vi "Register Step Handler.vi"(8 "error in (no error)":errorcluster, 10 "Handler":refnum<class "Handler.lvclass">, 11 "Server in":refnum<class "Server.lvclass">) -> (0 "error out":errorcluster, 3 "Server out":refnum<class "Server.lvclass">)   [LabVIEW 2020, in "HTTP Server.lvlib" / "Server.lvclass"]
uses:
  Server.lvclass
  Handler/Handler.lvclass
  Server.lvclass/Server.ctl
  Connection Handler/Connection Handler.lvclass
  Request Handler/Request Handler.lvclass
  Route Handler/Route Handler.lvclass
  Controller Handler/Controller Handler.lvclass
  Controller/Controller.lvclass
  Response Handler/Response Handler.lvclass
  Complete Handler/Complete Handler.lvclass
  Exception Handler/Exception Handler.lvclass
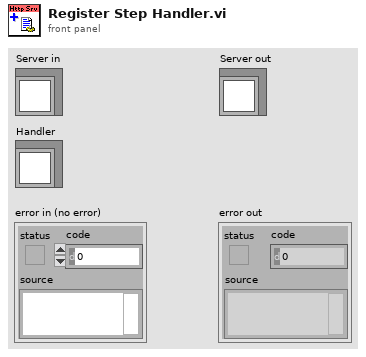
[diagram p1: front panel]
types:
  T1 = typedef "HTTP Server.lvlib/Processing Step.ctl" = enum16{"Connection", "Request", "Routing", "Controller Init", "Controller", "Response", "Cleanup", "Exception"}
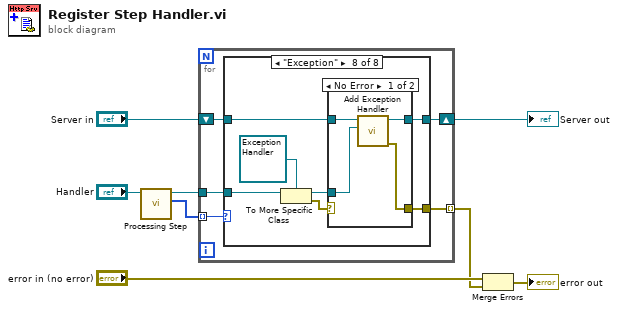
[diagram p0: block diagram]
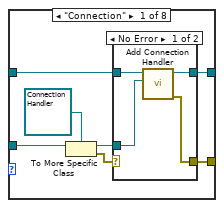
[diagram p2: hidden frame]
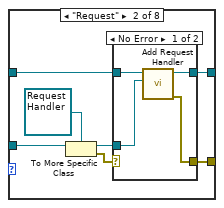
[diagram p4: hidden frame]
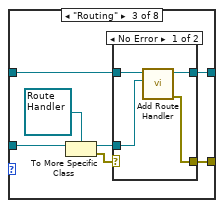
[diagram p6: hidden frame]
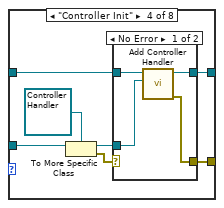
[diagram p8: hidden frame]
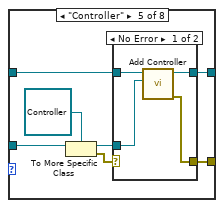
[diagram p10: hidden frame]
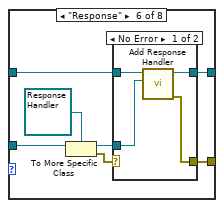
[diagram p12: hidden frame]
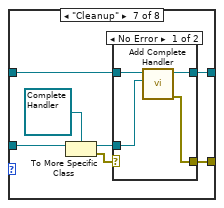
[diagram p14: hidden frame]
diagram:
  n1 = call-dynamic "Processing Step.vi"("Handler in"="Handler") -> ("Array"=w5:T1[], "Handler out"=w4:refnum<class "Handler.lvclass">)  [unwired: 8 in, 1 out]
  n2 = for {
    tunnel: w5 -> [w13] mode=indexing
    tunnel: w4 -> [w11]
    shift-right: [w10] -> w2
    shift-left: "Server in" -> [w12]
    tunnel: [w9] -> w1 mode=indexing
    n3 = case shown="\"Exception\"" w13 {
      tunnel: w12 -> [w16 w29 w42 w55 w68 w81 w94 w107]
      tunnel: w11 -> [w20 w33 w46 w59 w72 w85 w98 w111]
      tunnel: [w15 w28 w41 w54 w67 w80 w93 w106] -> w10
      tunnel: [w14 w27 w40 w53 w66 w79 w92 w105] -> w9
      frame "Connection" {
        n4 = To More Specific Class(target class=refnum<class "Connection Handler.lvclass"> refnum ("HTTP Server.lvlib:Connection Handler.lvclass"), reference=w20) -> (specific class reference=w18:refnum<class "Connection Handler.lvclass">, error out=w17:errorcluster)  [unwired: 1 in]
        n5 = case shown="No Error" w17 {
          selector: w17 -> [_ w26]
          tunnel: w18 -> [w23 _]
          tunnel: w16 -> [w24 w25]
          tunnel: [w22 w25] -> w15
          tunnel: [w21 w26] -> w14
          frame No Error {
            n6 = call "Add Connection Handler.vi"("Connection Handler"=w23, "Server in"=w24) -> ("error out"=w21:errorcluster, "Server out"=w22:refnum<class "Server.lvclass">)  [unwired: 8 in]
          }
          frame Error {
          }
        }
      }
      frame "Request" {
        n7 = To More Specific Class(target class=refnum<class "Request Handler.lvclass"> refnum ("HTTP Server.lvlib:Request Handler.lvclass"), reference=w33) -> (specific class reference=w31:refnum<class "Request Handler.lvclass">, error out=w30:errorcluster)  [unwired: 1 in]
        n8 = case shown="No Error" w30 {
          selector: w30 -> [_ w39]
          tunnel: w31 -> [w36 _]
          tunnel: w29 -> [w37 w38]
          tunnel: [w35 w38] -> w28
          tunnel: [w34 w39] -> w27
          frame No Error {
            n9 = call "Add Request Handler.vi"("Request Handler"=w36, "Server in"=w37) -> ("error out"=w34:errorcluster, "Server out"=w35:refnum<class "Server.lvclass">)  [unwired: 8 in]
          }
          frame Error {
          }
        }
      }
      frame "Routing" {
        n10 = To More Specific Class(target class=refnum<class "Route Handler.lvclass"> refnum ("HTTP Server.lvlib:Route Handler.lvclass"), reference=w46) -> (specific class reference=w44:refnum<class "Route Handler.lvclass">, error out=w43:errorcluster)  [unwired: 1 in]
        n11 = case shown="No Error" w43 {
          selector: w43 -> [_ w52]
          tunnel: w44 -> [w49 _]
          tunnel: w42 -> [w50 w51]
          tunnel: [w48 w51] -> w41
          tunnel: [w47 w52] -> w40
          frame No Error {
            n12 = call "Add Route Handler.vi"("Route Handler"=w49, "Server in"=w50) -> ("error out"=w47:errorcluster, "Server out"=w48:refnum<class "Server.lvclass">)  [unwired: 8 in]
          }
          frame Error {
          }
        }
      }
      frame "Controller Init" {
        n13 = To More Specific Class(target class=refnum<class "Controller Handler.lvclass"> refnum ("HTTP Server.lvlib:Controller Handler.lvclass"), reference=w59) -> (specific class reference=w57:refnum<class "Controller Handler.lvclass">, error out=w56:errorcluster)  [unwired: 1 in]
        n14 = case shown="No Error" w56 {
          selector: w56 -> [_ w65]
          tunnel: w57 -> [w62 _]
          tunnel: w55 -> [w63 w64]
          tunnel: [w61 w64] -> w54
          tunnel: [w60 w65] -> w53
          frame No Error {
            n15 = call "Add Controller Handler.vi"("Controller Handler"=w62, "Server in"=w63) -> ("error out"=w60:errorcluster, "Server out"=w61:refnum<class "Server.lvclass">)  [unwired: 8 in]
          }
          frame Error {
          }
        }
      }
      frame "Controller" {
        n16 = To More Specific Class(target class=refnum<class "Controller.lvclass"> refnum ("HTTP Server.lvlib:Controller.lvclass"), reference=w72) -> (specific class reference=w70:refnum<class "Controller.lvclass">, error out=w69:errorcluster)  [unwired: 1 in]
        n17 = case shown="No Error" w69 {
          selector: w69 -> [_ w78]
          tunnel: w70 -> [w75 _]
          tunnel: w68 -> [w76 w77]
          tunnel: [w74 w77] -> w67
          tunnel: [w73 w78] -> w66
          frame No Error {
            n18 = call "Add Controller.vi"("Controller"=w75, "Server in"=w76) -> ("error out"=w73:errorcluster, "Server out"=w74:refnum<class "Server.lvclass">)  [unwired: 8 in]
          }
          frame Error {
          }
        }
      }
      frame "Response" {
        n19 = To More Specific Class(target class=refnum<class "Response Handler.lvclass"> refnum ("HTTP Server.lvlib:Response Handler.lvclass"), reference=w85) -> (specific class reference=w83:refnum<class "Response Handler.lvclass">, error out=w82:errorcluster)  [unwired: 1 in]
        n20 = case shown="No Error" w82 {
          selector: w82 -> [_ w91]
          tunnel: w83 -> [w88 _]
          tunnel: w81 -> [w89 w90]
          tunnel: [w87 w90] -> w80
          tunnel: [w86 w91] -> w79
          frame No Error {
            n21 = call "Add Response Handler.vi"("Response Handler"=w88, "Server in"=w89) -> ("error out"=w86:errorcluster, "Server out"=w87:refnum<class "Server.lvclass">)  [unwired: 8 in]
          }
          frame Error {
          }
        }
      }
      frame "Cleanup" {
        n22 = To More Specific Class(target class=refnum<class "Complete Handler.lvclass"> refnum ("HTTP Server.lvlib:Complete Handler.lvclass"), reference=w98) -> (specific class reference=w96:refnum<class "Complete Handler.lvclass">, error out=w95:errorcluster)  [unwired: 1 in]
        n23 = case shown="No Error" w95 {
          selector: w95 -> [_ w104]
          tunnel: w96 -> [w101 _]
          tunnel: w94 -> [w102 w103]
          tunnel: [w100 w103] -> w93
          tunnel: [w99 w104] -> w92
          frame No Error {
            n24 = call "Add Complete Handler.vi"("Complete Handler"=w101, "Server in"=w102) -> ("error out"=w99:errorcluster, "Server out"=w100:refnum<class "Server.lvclass">)  [unwired: 8 in]
          }
          frame Error {
          }
        }
      }
      frame "Exception" {
        n25 = To More Specific Class(target class=refnum<class "Exception Handler.lvclass"> refnum ("HTTP Server.lvlib:Exception Handler.lvclass"), reference=w111) -> (specific class reference=w109:refnum<class "Exception Handler.lvclass">, error out=w108:errorcluster)  [unwired: 1 in]
        n26 = case shown="No Error" w108 {
          selector: w108 -> [_ w117]
          tunnel: w109 -> [w114 _]
          tunnel: w107 -> [w115 w116]
          tunnel: [w113 w116] -> w106
          tunnel: [w112 w117] -> w105
          frame No Error {
            n27 = call "Add Exception Handler.vi"("Exception Handler"=w114, "Server in"=w115) -> ("error out"=w112:errorcluster, "Server out"=w113:refnum<class "Server.lvclass">)  [unwired: 8 in]
          }
          frame Error {
          }
        }
      }
    }
  }
  "Server out" <- w2
  n28 = Merge Errors("error in (no error)", w1) -> (→"error out":errorcluster)
